vi "UHR-Fleezers Control (host) - 11.9.vi"() -> ()   [LabVIEW 2014] (continued)
            n1964 = Reshape Array(w2812, 3 ("dimension size")) -> (w2810:dbl[])
            n1965 = Array To Cluster(array=w2810) -> (cluster=w2809:cluster{"[0]":dbl, "[1]":dbl, "[2]":dbl})
            n1966 = call "Set Stage Position.vi"("Position"=w2809, "error in"=w2804, "VISA resource name in"=w2805) -> ("error out"=w2808:errorcluster)  [unwired: 2 out]
            n1967 = local write "Stage Moving"(TRUE ("Stage Moving")) -> ()
            n1968 = local write "Stage Control Serial Error"(w2808) -> ()
          }
          frame #1 {
            n1969 = local write "Stage Moving"(FALSE ("Stage Moving")) -> ()
            n1970 = call <vilib>:"Beep.vi"() -> ()  [unwired: 3 in, 9 out]
          }
        }
      }
      event "Set Current\nPos to 0,0,0": Value Change {
        # "DH is \"Define Home\""
        n1971 = event-data() -> ()  [unwired: 1 in, 6 out]
        n1972 = local write "Set Current\nPos to 0,0,0"(FALSE ("Set Current\nPos to 0,0,0")) -> ()
        n1973 = Concatenate Strings("1DH" ("string"), ";" ("string"), "2DH" ("string"), ";" ("string"), "3DH" ("string"), "\r") -> (w2823:string)
        n1974 = call-poly "VISA Configure Serial Port"("VISA resource name"=w2828, "baud rate (9600)"=u32 19200, "error in (no error)"=w2827) -> ("VISA resource name out"=w2825:refnum<visa-resource-name>, "error out"=w2824:errorcluster)  [unwired: 11 in]
        n1975 = VISA Write(VISA resource name=w2825, write buffer=w2823, error in (no error)=w2824) -> (error out=w2818:errorcluster)  [unwired: 2 out]
        n1976 = local write "Stage Control Serial Error"(w2818) -> ()
      }
      event "Got ADig bead": Value Change {
        n1977 = event-data() -> ()  [unwired: 1 in, 5 out]
        n1978 = flat-sequence {
          frame #0 {
            n1979 = local read "Cap 1 Samp Flow ON"() -> (w2833:bool)
            n1980 = case shown="True" w2833 {
              frame False {
              }
              frame True {
                n1981 = property on="Sample Channel\nFlow" class="Bool (strict)"("Val(Sgnl)"=TRUE ("Value (Signaling)")) -> ()  [unwired: 2 in, 2 out]
              }
            }
          }
          frame #1 {
            n1982 = property on="Inject Pump 3" class="Bool (strict)"("Val(Sgnl)"=FALSE ("Value (Signaling)")) -> ()  [unwired: 2 in, 2 out]
            n1983 = local write "Target"(FALSE ("Target")) -> ()
          }
          frame #2 {
            n1984 = property on="Move Cap. 1 (DNA Bottom)" class="Bool (strict)"("Val(Sgnl)"=TRUE ("Value (Signaling)")) -> ()  [unwired: 2 in, 2 out]
          }
        }
      }
      event "Force FB Script": Value Change {
        n1985 = event-data() -> ()  [unwired: 1 in, 5 out]
        n1986 = local write "Force FB Script"(FALSE ("Force FB Data\nScript")) -> ()
        n1987 = flat-sequence {
          tunnel: w2844 -> [w2848]
          tunnel: w2845 -> [w2849]
          tunnel: [w2849] -> w2840
          tunnel: [w2848] -> w2839
          tunnel: w2840 -> [w2852]
          tunnel: w2839 -> [w2851]
          tunnel: ["Trap Trig Fl."] -> w2841
          tunnel: [w2894] -> w2842
          tunnel: w2841 -> [w2894]
          tunnel: [w2898] -> w2843
          tunnel: w2842 -> [w2898]
          tunnel: w2843 -> [w2900]
          frame #0 {
            n1988 = property on="Trap D (MHz)" class="DigNum (strict)"("Val(Sgnl)"="Trap D Before Moving") -> ()  [unwired: 2 in, 2 out]
          }
          frame #1 {
            n1989 = local read "Saved Stage Positions"() -> (w2854:dbl[][])
            n1990 = local write "FB Trap Pos Offset"(0.0 ("FB Trap Pos Offset")) -> ()
            n1991 = property on="Trap Pos. FB Offset Factor" class="DigNum (strict)"("Val(Sgnl)"=i64 0 ("Value (Signaling)")) -> ()  [unwired: 2 in, 2 out]
            n1992 = local write "Stage Moving"(TRUE ("Stage Moving")) -> ()
            n1993 = call "move to saved stage position.vi"("error in"=w2851, "Stage VISA resource name in"=w2852, "Position"="Stage Position To Establish FB", "Saved Stage Positions"=w2854) -> ("error out"=w2850:errorcluster)  [unwired: 1 out]
            n1994 = local write "Stage Control Serial Error"(w2850) -> ()
          }
          frame #2 {
            n1995 = call <vilib>:"Beep.vi"("duration (msec)"=u32 100, "frequency (Hz)"=u32 20) -> ()  [unwired: 1 in, 9 out]
            n1996 = local write "Stage Moving"(FALSE ("Stage Moving")) -> ()
            n1997 = property on="Tab Control 2" class="TabCtl (strict)"("Val(Sgnl)"=T6."Feedback on Trap Position" ("Value (Signaling)")) -> ()  [unwired: 2 in, 2 out]
            n1998 = stacked-sequence {
              frame #0 {
                n1999 = Multiply(x="Wait (s)", y=u32 1000 ("milliseconds to wait")) -> (x*y=w2863:u32)
                n2000 = property on="Trap D (MHz)" class="DigNum (strict)"("Val(Sgnl)"="Starting Trap D (MHz)") -> ()  [unwired: 2 in, 2 out]
                n2001 = Wait (ms)(milliseconds to wait=w2863) -> ()  [unwired: 1 out]
              }
              frame #1 {
                n2002 = property on="Set Reading to\nSetpoint" class="Bool (strict)"("Val(Sgnl)"=TRUE ("Value (Signaling)")) -> ()  [unwired: 2 in, 2 out]
              }
            }
            n2003 = property on="Tab Control" class="TabCtl (strict)"("Val(Sgnl)"=T4."Trap Control (RF)" ("Value (Signaling)")) -> ()  [unwired: 2 in, 2 out]
          }
          frame #3 {
            n2004 = Wait (ms)(milliseconds to wait=u32 500) -> ()  [unwired: 1 out]
          }
          frame #4 {
            n2005 = property on="Trap Pos. FB ON" class="Bool (strict)"("Val(Sgnl)"=TRUE ("Value (Signaling)")) -> ()  [unwired: 2 in, 2 out]
            n2006 = Wait (ms)(milliseconds to wait=u32 250) -> ()  [unwired: 1 out]
          }
          frame #5 {
            n2007 = case shown="\"1\"" "Remove Action Offset Dropdown" {
              tunnel: TRUE ("Value (Signaling)") -> [w2875 w2883 w2891]
              frame "1" {
                n2008 = flat-sequence {
                  tunnel: w2875 -> [w2882]
                  frame #0 {
                    n2009 = local read "factor"() -> (w2877:dbl)
                    n2010 = Greater Than 0?(x=w2877) -> (x > 0?=w2881:bool)
                    n2011 = Select(t=1.0, s=w2881, f=-1.0) -> (s? t:f=w2878:dbl)
                    n2012 = Multiply(x=w2878, y=w2877) -> (x*y=w2876:dbl)
                    n2013 = local write "factor"(w2876) -> ()
                  }
                  frame #1 {
                    n2014 = property on="Remove Offset to factor" class="Bool (strict)"("Val(Sgnl)"=w2882) -> ()  [unwired: 2 in, 2 out]
                  }
                }
              }
              frame "2" {
                n2015 = flat-sequence {
                  tunnel: w2883 -> [w2890]
                  frame #0 {
                    n2016 = local read "factor"() -> (w2884:dbl)
                    n2017 = Greater Than 0?(x=w2884) -> (x > 0?=w2889:bool)
                    n2018 = Select(t=-1.0, s=w2889, f=1.0) -> (s? t:f=w2887:dbl)
                    n2019 = Multiply(x=w2884, y=w2887) -> (x*y=w2886:dbl)
                    n2020 = local write "factor"(w2886) -> ()
                  }
                  frame #1 {
                    n2021 = property on="Remove Offset to factor" class="Bool (strict)"("Val(Sgnl)"=w2890) -> ()  [unwired: 2 in, 2 out]
                  }
                }
              }
              frame "0", Default {
                n2022 = property on="Remove Action Offset" class="Bool (strict)"("Val(Sgnl)"=w2891) -> ()  [unwired: 2 in, 2 out]
              }
            }
            n2023 = case shown="False" "Trap Trig Fl." {
              frame False {
                n2024 = case shown="True" "Green ON after FB ON?" {
                  selector: "Green ON after FB ON?" -> [_ w2893]
                  frame False {
                  }
                  frame True {
                    n2025 = property on="Green ON/Interlacing" class="Bool (strict)"("Val(Sgnl)"=w2893) -> ()  [unwired: 2 in, 2 out]
                  }
                }
              }
              frame True {
              }
            }
            n2026 = Wait (ms)(milliseconds to wait=u32 250) -> ()  [unwired: 1 out]
          }
          frame #6 {
            n2027 = property on="Start Saving" class="Bool (strict)"("Val(Sgnl)"=TRUE ("Value (Signaling)")) -> ()  [unwired: 2 in, 2 out]
            n2028 = Wait (ms)(milliseconds to wait=u32 5000) -> ()  [unwired: 1 out]
          }
          frame #7 {
            w2897 = TRUE ("Value (Signaling)")
            n2029 = property on="Rem fb disp offset" class="Bool (strict)"("Val(Sgnl)"=w2897) -> ()  [unwired: 2 in, 2 out]
            n2030 = property on="Remove Offset" class="Bool (strict)"("Val(Sgnl)"=w2897) -> ()  [unwired: 2 in, 2 out]
            n2031 = Wait (ms)(milliseconds to wait=u32 100) -> ()  [unwired: 1 out]
          }
          frame #8 {
            n2032 = case shown="True" w2900 {
              frame False {
              }
              frame True {
                n2033 = local write "Trap Trig. Fl."(TRUE ("Value (Signaling)")) -> ()
              }
            }
          }
          frame #9 {
            n2034 = local read "Tether"() -> (w2903:bool)
            n2035 = And(x="Start dipping after?", y=w2903) -> (x .and. y?=w2902:bool)
            n2036 = case shown="True" w2902 {
              frame False {
              }
              frame True {
                n2037 = flat-sequence {
                  frame #0 {
                    n2038 = Multiply(x="Delay before dipping (s)", y=1000.0) -> (x*y=w2906:dbl)
                    n2039 = Wait (ms)(milliseconds to wait=w2906) -> ()  [unwired: 1 out]
                  }
                  frame #1 {
                    n2040 = property on="Dip for Protein" class="Bool (strict)"("Val(Sgnl)"=TRUE ("Value (Signaling)")) -> ()  [unwired: 2 in, 2 out]
                    n2041 = local write "Scripts"(T29."Dipping") -> ()
                  }
                }
              }
            }
          }
        }
      }
      event "Rupture Script": Value Change {
        n2042 = event-data() -> ()  [unwired: 1 in, 5 out]
        n2043 = local write "Rupture Script"(FALSE ("Rupture Script")) -> ()
        n2044 = flat-sequence {
          frame #0 {
            w2912 = TRUE
            w2917 = FALSE
            # "Number 6 for now is the\nrupture-experiment\nparameters."
            n2045 = local read "Starting Trap D (MHz)"() -> (w2918:dbl)
            n2046 = local write "Restart DMA? (AOD)"(w2917) -> ()
            n2047 = Replace Array Subset(array=u32[] [0] ("Index Values"), new element=6, index=0) -> (w2913:u32[])
            n2048 = local write "Save scans"(w2917) -> ()
            n2049 = property on="Trap D (MHz)" class="DigNum (strict)"("Val(Sgnl)"=w2918) -> ()  [unwired: 2 in, 2 out]
            n2050 = property on="Saved AOD Raster Scan Parameter Sets" class="Arr (strict)"("Index Values"=w2913) -> ()  [unwired: 2 in, 2 out]
            n2051 = property on="Start Saving" class="Bool (strict)"("Val(Sgnl)"=w2912) -> ()  [unwired: 2 in, 2 out]
            n2052 = property on="Green ON/Interlacing" class="Bool (strict)"("Val(Sgnl)"=w2912) -> ()  [unwired: 2 in, 2 out]
          }
          frame #1 {
            n2053 = property on="Load parameters" class="Bool (strict)"("Val(Sgnl)"=TRUE ("Value (Signaling)")) -> ()  [unwired: 2 in, 2 out]
          }
        }
      }
      event "Fixed Traps Script": Value Change {
        n2054 = event-data() -> ()  [unwired: 1 in, 5 out]
        n2055 = local write "Fixed Traps Script"(FALSE ("Fixed Traps Data\nScript")) -> ()
        n2056 = flat-sequence {
          frame #0 {
            n2057 = case shown="True" "Green ON" {
              frame False {
              }
              frame True {
                n2058 = property on="Green ON/Interlacing" class="Bool (strict)"("Val(Sgnl)"=TRUE) -> ()  [unwired: 2 in, 2 out]
              }
            }
            n2059 = local write "Offset (nm)"(0.0 ("Offset (nm)")) -> ()
            n2060 = property on="Sample Channel\nFlow" class="Bool (strict)"("Val(Sgnl)"=FALSE ("Value (Signaling)")) -> ()  [unwired: 2 in, 2 out]
            n2061 = property on="Trap D (MHz)" class="DigNum (strict)"("Val(Sgnl)"="Fixed Traps Trap Delta (MHz)") -> ()  [unwired: 2 in, 2 out]
          }
          frame #1 {
            n2062 = Wait (ms)(milliseconds to wait=u32 1000) -> ()  [unwired: 1 out]
          }
          frame #2 {
            n2063 = local write "Start Saving"(TRUE ("Start Saving")) -> ()
          }
          frame #3 {
            n2064 = local read "Bead Sep. Int. Time (s)"() -> (w2928:dbl)
            n2065 = Multiply(x=w2928, y=1000.0) -> (x*y=w2930:dbl)
            n2066 = Wait (ms)(milliseconds to wait=w2930) -> ()  [unwired: 1 out]
          }
          frame #4 {
            n2067 = property on="Remove Offset" class="Bool (strict)"("Val(Sgnl)"=TRUE ("Value (Signaling)")) -> ()  [unwired: 2 in, 2 out]
          }
          frame #5 {
            n2068 = property on="Dip for Protein" class="Bool (strict)"("Val(Sgnl)"="Start dipping after?") -> ()  [unwired: 2 in, 2 out]
          }
        }
      }
      event "Got DNA bead": Value Change {
        n2069 = event-data() -> ()  [unwired: 1 in, 5 out]
        n2070 = flat-sequence {
          frame #0 {
            n2071 = local read "Daq spot flow on"() -> (w2935:bool)
            n2072 = case shown="True" w2935 {
              frame False {
              }
              frame True {
                n2073 = property on="Sample Channel\nFlow" class="Bool (strict)"("Val(Sgnl)"=TRUE ("Value (Signaling)")) -> ()  [unwired: 2 in, 2 out]
              }
            }
            n2074 = property on="Got DNA bead" class="Bool"("Key Focus"=FALSE) -> ()  [unwired: 2 in, 2 out]
          }
          frame #1 {
            n2075 = property on="Inject Pump 1" class="Bool (strict)"("Val(Sgnl)"=FALSE ("Value (Signaling)")) -> ()  [unwired: 2 in, 2 out]
          }
          frame #2 {
            n2076 = property on="Cal/Data Acq. Spot" class="Bool (strict)"("Val(Sgnl)"=TRUE ("Value (Signaling)")) -> ()  [unwired: 2 in, 2 out]
          }
        }
      }
      event "Take Stepping Data": Value Change {
        n2077 = event-data() -> ()  [unwired: 1 in, 5 out]
        n2078 = local read "Save ave N"() -> (w2947:dbl)
        n2079 = flat-sequence {
          tunnel: w2947 -> [w2949]
          tunnel: [w2949] -> w2942
          tunnel: [w2951] -> w2943
          tunnel: w2942 -> [w2951]
          tunnel: [w2953] -> w2944
          tunnel: w2943 -> [w2953]
          tunnel: [w2956] -> w2945
          tunnel: w2944 -> [w2956]
          tunnel: [w2958] -> w2946
          tunnel: w2945 -> [w2958]
          tunnel: [w2960] -> w2940
          tunnel: w2946 -> [w2960]
          tunnel: w2940 -> [w2963]
          tunnel: [w2963] -> w2939
          tunnel: w2939 -> [w2964]
          tunnel: [w2964] -> w2941
          tunnel: w2941 -> [w2970]
          frame #0 {
            n2080 = property on="Save ave N" class="DigNum (strict)"("Val(Sgnl)"="Save ave factor") -> ()  [unwired: 2 in, 2 out]
          }
          frame #1 {
            n2081 = Wait (ms)(milliseconds to wait=u32 100) -> ()  [unwired: 1 out]
          }
          frame #2 {
            n2082 = local read "Offset 2 Start (MHz)"() -> (w2955:dbl)
            n2083 = property on="Saved AOD Raster Scan Parameter Sets" class="Arr (strict)"("Index Values"=u32[] [2]) -> ()  [unwired: 2 in, 2 out]
            n2084 = property on="Trap D (MHz)" class="DigNum (strict)"("Val(Sgnl)"=w2955) -> ()  [unwired: 2 in, 2 out]
          }
          frame #3 {
            n2085 = property on="Load parameters" class="Bool (strict)"("Val(Sgnl)"=TRUE ("Value (Signaling)")) -> ()  [unwired: 2 in, 2 out]
          }
          frame #4 {
            n2086 = Wait (ms)(milliseconds to wait=u32 100) -> ()  [unwired: 1 out]
          }
          frame #5 {
            n2087 = property on="Trap Raster Scan" class="Bool (strict)"("Val(Sgnl)"=TRUE ("Value (Signaling)")) -> ()  [unwired: 2 in, 2 out]
          }
          frame #6 {
            n2088 = Wait (ms)(milliseconds to wait=u32 1000) -> ()  [unwired: 1 out]
          }
          frame #7 {
            n2089 = while {
              stop <- w2967 stop-if-true
              n2090 = local read "Raster Scanning..."() -> (w2969:bool)
              n2091 = local read "Saving..."() -> (w2968:bool)
              n2092 = Not(x=w2968) -> (.not. x?=w2965:bool)
              n2093 = Not(x=w2969) -> (.not. x?=w2966:bool)
              n2094 = And(x=w2966, y=w2965) -> (x .and. y?=w2967:bool)
            }
          }
          frame #8 {
            n2095 = property on="Save ave N" class="DigNum (strict)"("Val(Sgnl)"=w2970) -> ()  [unwired: 2 in, 2 out]
          }
        }
      }
      event "Step Size (nm)": Value Change {
        n2096 = event-data() -> ()  [unwired: 1 in, 5 out]
        n2097 = flat-sequence {
          frame #0 {
            n2098 = property on="Saved AOD Raster Scan Parameter Sets" class="Arr (strict)"("Index Values"=u32[] [1]) -> ()  [unwired: 2 in, 2 out]
          }
          frame #1 {
            n2099 = Multiply(x="N Steps", y="Step Size (nm)") -> (x*y=w2972:dbl)
            n2100 = property on="Scan Speed AOD (nm/s) 2" class="DigNum (strict)"("Value"="Step Size (nm)") -> ()  [unwired: 2 in, 2 out]
            n2101 = property on="Step Size AOD (nm) 2" class="DigNum (strict)"("Value"="Step Size (nm)") -> ()  [unwired: 2 in, 2 out]
            n2102 = property on="Scan Range AOD (nm) 2" class="DigNum (strict)"("Value"=w2972) -> ()  [unwired: 2 in, 2 out]
          }
        }
      }
      event "Take Detection Laser\nImage": Value Change {
        n2103 = event-data() -> ()  [unwired: 1 in, 5 out]
        n2104 = flat-sequence {
          tunnel: [w3000] -> w2990
          tunnel: [w2999] -> w2983
          tunnel: [w2998] -> w2975
          tunnel: [w3003] -> w2991
          tunnel: w2990 -> [w3003]
          tunnel: [w3002] -> w2984
          tunnel: w2983 -> [w3002]
          tunnel: [w3001] -> w2976
          tunnel: w2975 -> [w3001]
          tunnel: [w3007] -> w2992
          tunnel: w2991 -> [w3007]
          tunnel: [w3006] -> w2985
          tunnel: w2984 -> [w3006]
          tunnel: [w3005] -> w2977
          tunnel: w2976 -> [w3005]
          tunnel: [w3013] -> w2993
          tunnel: w2992 -> [w3013]
          tunnel: [w3012] -> w2986
          tunnel: w2985 -> [w3012]
          tunnel: [w3011] -> w2978
          tunnel: w2977 -> [w3011]
          tunnel: [w3017] -> w2994
          tunnel: w2993 -> [w3017]
          tunnel: [w3016] -> w2987
          tunnel: w2986 -> [w3016]
          tunnel: [w3015] -> w2979
          tunnel: w2978 -> [w3015]
          tunnel: [w3021] -> w2995
          tunnel: w2994 -> [w3021]
          tunnel: [w3020] -> w2988
          tunnel: w2987 -> [w3020]
          tunnel: [w3019] -> w2980
          tunnel: w2979 -> [w3019]
          tunnel: [w3025] -> w2996
          tunnel: w2995 -> [w3025]
          tunnel: [w3024] -> w2989
          tunnel: w2988 -> [w3024]
          tunnel: [w3023] -> w2981
          tunnel: w2980 -> [w3023]
          tunnel: w2996 -> [w3031]
          tunnel: w2989 -> [w3030]
          tunnel: [w3028] -> w2982
          tunnel: w2981 -> [w3028]
          tunnel: w2982 -> [w3032]
          frame #0 {
            n2105 = local read "Green ON/Interlacing"() -> (w3000:bool)
            n2106 = local read "Green laser mode"() -> (w2999:enum32{"Laser ON", "Laser OFF", "Interlace"})
            n2107 = local read "Green FB On/Off"() -> (w2998:bool)
          }
          frame #1 {
            n2108 = property on="Green FB On/Off" class="Bool (strict)"("Val(Sgnl)"=FALSE ("Value (Signaling)")) -> ()  [unwired: 2 in, 2 out]
          }
          frame #2 {
            n2109 = property on="Green ON/Interlacing" class="Bool (strict)"("Val(Sgnl)"=TRUE ("Value (Signaling)")) -> ()  [unwired: 2 in, 2 out]
            n2110 = property on="Flip Green Filter" class="Bool (strict)"("Val(Sgnl)"=TRUE ("Value (Signaling)")) -> ()  [unwired: 2 in, 2 out]
            n2111 = property on="Green laser mode" class="RadioBtnsControl (strict)"("Val(Sgnl)"=enum32{"Laser ON", "Laser OFF", "Interlace"}."Laser ON" ("Value (Signaling)")) -> ()  [unwired: 2 in, 2 out]
          }
          frame #3 {
            n2112 = Wait (ms)(milliseconds to wait=u32 500) -> ()  [unwired: 1 out]
          }
          frame #4 {
            n2113 = property on="Confocal\nImage" class="Bool (strict)"("Val(Sgnl)"=TRUE ("Value (Signaling)")) -> ()  [unwired: 2 in, 2 out]
          }
          frame #5 {
            n2114 = Wait (ms)(milliseconds to wait=u32 2000) -> ()  [unwired: 1 out]
          }
          frame #6 {
            n2115 = while {
              stop <- w3026 stop-if-true
              n2116 = local read "Saving..."() -> (w3027:bool)
              n2117 = Not(x=w3027) -> (.not. x?=w3026:bool)
            }
          }
          frame #7 {
            n2118 = property on="Flip Green Filter" class="Bool (strict)"("Val(Sgnl)"=TRUE ("Value (Signaling)")) -> ()  [unwired: 2 in, 2 out]
            n2119 = property on="Green ON/Interlacing" class="Bool (strict)"("Val(Sgnl)"=w3031) -> ()  [unwired: 2 in, 2 out]
            n2120 = property on="Green laser mode" class="RadioBtnsControl (strict)"("Val(Sgnl)"=w3030) -> ()  [unwired: 2 in, 2 out]
          }
          frame #8 {
            n2121 = property on="Green FB On/Off" class="Bool (strict)"("Val(Sgnl)"=w3032) -> ()  [unwired: 2 in, 2 out]
          }
        }
      }
      event "Stop All": Value Change {
        n2122 = event-data() -> ()  [unwired: 1 in, 5 out]
        n2123 = local read "Stop All"() -> (w3033:bool)
      }
    }
    n2124 = node-c288() -> ()  [unwired: 1 in, 1 out]
  }
  n2125 = node-c288() -> (w112:T21)  [unwired: 4 out]
  n2126 = timed-loop "Mouse control: trap position (AOM deflection), set confocal spot from image" {
    tunnel: [w3035] -> w200
    tunnel: w20 -> [w3034]
    timing: w112 -> [_]
    timing-out: [_] -> w111
    stop <- w3035 stop-if-true
    n2127 = node-c288() -> ()  [unwired: 2 out]
    n2128 = event shown="[0] \"Pane\": Mouse Down" {
      selector: _ -> [_ _]
      dyn-events: _ -> [_ _]
      timeout: _ -> [_ _]
      tunnel: w3034 -> [w3038 _]
      event Mouse Down {
        n2129 = event-data() -> ("Time"=w3040:u32, "Coords"=w3039:T7, "Button"=w3041:u16)  [unwired: 6 out]
        n2130 = case shown="1" w3041 {
          tunnel: w3040 -> [_ _ w3180]
          tunnel: w3039 -> [_ w3046 w3178]
          tunnel: w3038 -> [_ _ w3176]
          frame 0, Default {
          }
          frame 1 {
            n2131 = property on="APD 2" class="ImageControl"() -> ("Displayed Image Position"=w3060:cluster{"Left":i32, "Top":i32})  [unwired: 2 in, 2 out]
            n2132 = control-ref of="Primary Video Display"() -> (w3053:refnum<vi>)
            n2133 = property on="APD 1" class="ImageControl"() -> ("Displayed Image Position"=w3089:cluster{"Left":i32, "Top":i32})  [unwired: 2 in, 2 out]
            n2134 = property on="Detection Laser X" class="ImageControl"() -> ("Displayed Image Position"=w3086:cluster{"Left":i32, "Top":i32})  [unwired: 2 in, 2 out]
            n2135 = property on="Detection Laser Y" class="ImageControl"() -> ("Displayed Image Position"=w3085:cluster{"Left":i32, "Top":i32})  [unwired: 2 in, 2 out]
            n2136 = property on="APD 2" class="ImageControl"() -> ("Displayed Image Size"=w3059:cluster{"Width":u32, "Height":u32})  [unwired: 2 in, 2 out]
            n2137 = property on="APD 1" class="ImageControl"() -> ("Displayed Image Size"=w3087:cluster{"Width":u32, "Height":u32})  [unwired: 2 in, 2 out]
            n2138 = property on="Detection Laser X" class="ImageControl"() -> ("Displayed Image Size"=w3088:cluster{"Width":u32, "Height":u32})  [unwired: 2 in, 2 out]
            n2139 = property on="Detection Laser Y" class="ImageControl"() -> ("Displayed Image Size"=w3084:cluster{"Width":u32, "Height":u32})  [unwired: 2 in, 2 out]
            n2140 = property class="ImageControl"(reference=w3053) -> ("Displayed Image Position"=w3051:cluster{"Left":i32, "Top":i32})  [unwired: 1 in, 2 out]
            n2141 = property class="ImageControl"(reference=w3053) -> ("Displayed Image Size"=w3052:cluster{"Width":u32, "Height":u32})  [unwired: 1 in, 2 out]
            n2142 = Unbundle By Name(w3059) -> ("Width"=w3056:u32, "Height"=w3055:u32)
            n2143 = Unbundle By Name(w3060) -> ("Left"=w3058:i32, "Top"=w3057:i32)
            n2144 = Unbundle By Name(w3087) -> ("Width"=w3081:u32, "Height"=w3080:u32)
            n2145 = Unbundle By Name(w3088) -> ("Width"=w3077:u32, "Height"=w3076:u32)
            n2146 = Unbundle By Name(w3084) -> ("Width"=w3073:u32, "Height"=w3072:u32)
            n2147 = Unbundle By Name(w3089) -> ("Left"=w3083:i32, "Top"=w3082:i32)
            n2148 = Unbundle By Name(w3086) -> ("Left"=w3079:i32, "Top"=w3078:i32)
            n2149 = Unbundle By Name(w3085) -> ("Left"=w3075:i32, "Top"=w3074:i32)
            n2150 = Bundle("Left"=w3058, "Top"=w3057, "Width"=w3056, "Height"=w3055) -> (w3054:T30)  [unwired: 1 in]
            n2151 = Bundle("Left"=w3083, "Top"=w3082, "Width"=w3081, "Height"=w3080) -> (w3071:T30)  [unwired: 1 in]
            n2152 = Bundle("Left"=w3079, "Top"=w3078, "Width"=w3077, "Height"=w3076) -> (w3070:T30)  [unwired: 1 in]
            n2153 = Bundle("Left"=w3075, "Top"=w3074, "Width"=w3073, "Height"=w3072) -> (w3069:T30)  [unwired: 1 in]
            n2154 = Unbundle By Name(w3052) -> ("Width"=w3048:u32, "Height"=w3047:u32)
            n2155 = Unbundle By Name(w3051) -> ("Left"=w3050:i32, "Top"=w3049:i32)
            n2156 = Build Cluster Array(w3054, w3071, w3070, w3069) -> (w3068:T31)
            n2157 = Bundle("Left"=w3050, "Top"=w3049, "Width"=w3048, "Height"=w3047) -> (w3043:T30)  [unwired: 1 in]
            n2158 = for {
              tunnel: w3046 -> [w3122]
              tunnel: w3068 -> [w3123] mode=indexing
              shift-right: [w3120] -> w3066
              shift-left: TRUE -> [w3121]
              shift-right: [w3119] -> w3064
              shift-left: _ -> [w3115]
              shift-right: [w3118] -> w3063
              shift-left: _ -> [w3114]
              shift-right: [w3117] -> w3062
              shift-left: _ -> [w3113]
              shift-right: [w3116] -> w3061
              shift-left: _ -> [w3112]
              n2159 = case shown="True" w3121 {
                selector: w3121 -> [w3128 _]
                tunnel: w3123 -> [_ w3137]
                tunnel: w3122 -> [_ w3135]
                tunnel: [w3128 w3133] -> w3120
                tunnel: [w3127 w3132] -> w3119
                tunnel: [w3126 w3131] -> w3118
                tunnel: [w3125 w3130] -> w3117
                tunnel: [w3124 w3129] -> w3116
                tunnel: w3115 -> [w3127 _]
                tunnel: w3114 -> [w3126 _]
                tunnel: w3113 -> [w3125 _]
                tunnel: w3112 -> [w3124 _]
                frame False {
                }
                frame True {
                  n2160 = Unbundle(w3137) -> (w3136:T30)
                  n2161 = call "isclickinwindow.vi"("Image Param"=w3136, "Point32"=w3135) -> ("4 Y"=w3129:i32, "3 Height"=w3130:i32, "2 X"=w3131:i32, "1 Width"=w3132:i32, "In image?"=w3134:bool)  [unwired: 1 in]
                  n2162 = Not(x=w3134) -> (.not. x?=w3133:bool)
                }
              }
            }
            n2163 = call "isclickinwindow.vi"("Image Param"=w3043, "Point32"=w3046) -> ("4 Y"=w3044:i32, "2 X"=w3045:i32, "In image?"=w3042:bool)  [unwired: 1 in, 2 out]
            n2164 = case shown="True" w3042 {
              tunnel: w3045 -> [_ w3093]
              tunnel: w3044 -> [_ w3096]
              frame False {
              }
              frame True {
                w3105 = 2
                n2165 = Subtract(x=480, y=w3096) -> (x-y=w3095:i32)
                n2166 = Unbundle("Target size") -> ("Width"=w3106:dbl, "Height"=w3104:dbl)
                n2167 = Subtract(x=w3093, y=2) -> (x-y=w3092:i32)
                n2168 = Divide(x=w3104, y=w3105) -> (x/y=w3102:dbl)
                n2169 = Divide(x=w3106, y=w3105) -> (x/y=w3103:dbl)
                n2170 = Subtract(x=w3092, y=w3103) -> (x-y=w3101:dbl)
                n2171 = Add(x=w3092, y=w3103) -> (x+y=w3099:dbl)
                n2172 = Subtract(x=w3095, y=w3102) -> (x-y=w3100:dbl)
                n2173 = Add(x=w3095, y=w3102) -> (x+y=w3098:dbl)
                n2174 = Bundle(w3092, w3095) -> (w3108:cluster{i32, i32})  [unwired: 1 in]
                n2175 = Bundle(w3101, w3100, w3099, w3098) -> (w3090:cluster{dbl, dbl, dbl, dbl})  [unwired: 1 in]
                n2176 = case shown="True" "Set target" {
                  tunnel: w3108 -> [_ w3111]
                  tunnel: w3090 -> [_ w3109]
                  frame False {
                  }
                  frame True {
                    n2177 = local write "Target coordinates"(w3109) -> ()
                    n2178 = local write "Set target"(FALSE ("Set target")) -> ()
                    "Video coordinates" <- w3111
                  }
                }
              }
            }
            n2179 = Not(x=w3066) -> (.not. x?=w3065:bool)
            n2180 = case shown="True" w3065 {
              tunnel: w3063 -> [_ w3151]
              tunnel: w3061 -> [_ w3150]
              tunnel: w3064 -> [_ w3149]
              tunnel: w3062 -> [_ w3148]
              frame False {
              }
              frame True {
                w3138 = FALSE ("Get Point")
                n2181 = local read "Scan lines (y)"() -> (w3153:u64)
                n2182 = disable-structure shown="Disabled" {
                  frame Disabled {
                  }
                  frame Enabled {
                  }
                }
                n2183 = local read "Actual MCL Inc (V)"() -> (w3147:dbl)
                n2184 = local read "Scan steps (MCL)"() -> (w3152:u64)
                n2185 = Divide "Y Pix/step"(x=w3148, y=w3153) -> (x/y=w3160:dbl)
                n2186 = Divide "Y V/pix"(x=w3147, y=w3160) -> (x/y=w3159:dbl)
                n2187 = Divide "Y half step offset"(x=w3147, y=2.0) -> (x/y=w3161:dbl)
                n2188 = Divide "X pix/step"(x=w3149, y=w3152) -> (x/y=w3158:dbl)
                n2189 = Negate(x=w3161) -> (-x=w3162:dbl)
                n2190 = local read "Initial Y"() -> (w3168:dbl)
                n2191 = Multiply(x=w3150, y=w3159) -> (x*y=w3169:dbl)
                n2192 = Divide "X half step offset"(x=w3147, y=2.0) -> (x/y=w3155:dbl)
                n2193 = Divide "X V/pix"(x=w3147, y=w3158) -> (x/y=w3157:dbl)
                n2194 = Multiply(x=w3147, y=w3152) -> (x*y=w3164:dbl)
                n2195 = Compound Arithmetic op=ADD(w3162, w3169, w3168) -> (w3139:dbl)
                "Pointer Y (V)" <- w3139
                n2196 = Multiply(x=w3157, y=w3151) -> (x*y=w3166:dbl)
                n2197 = Negate(x=w3155) -> (-x=w3154:dbl)
                n2198 = local read "Initial X"() -> (w3167:dbl)
                n2199 = Negate(x=w3166) -> (-x=w3165:dbl)
                n2200 = Compound Arithmetic op=ADD(w3154, w3164, w3167, w3165) -> (w3140:dbl)
                "Pointer X (V)" <- w3140
                n2201 = case shown="True" "Set High F Confocal Spot (X-Y)" {
                  tunnel: w3140 -> [_ w3170]
                  tunnel: w3139 -> [_ w3171]
                  frame False {
                  }
                  frame True {
                    "Confocal Y 2 (V)" <- w3171
                    "Confocal X 2 (V)" <- w3170
                  }
                }
                n2202 = Or(x="Set X Only", y="Set Confocal Spot (X-Y)") -> (x .or. y?=w3143:bool)
                n2203 = Or(x="Set Confocal Spot (X-Y)", y="Set Y Only") -> (x .or. y?=w3142:bool)
                n2204 = case shown="True" w3143 {
                  tunnel: w3140 -> [_ w3172]
                  frame False {
                  }
                  frame True {
                    n2205 = property on="AO2" class="Slide (strict)"("Val(Sgnl)"=w3172) -> ()  [unwired: 2 in, 2 out]
                    "Confocal X 1 (V)" <- w3172
                  }
                }
                n2206 = case shown="True" w3142 {
                  tunnel: w3139 -> [_ w3173]
                  frame False {
                  }
                  frame True {
                    n2207 = property on="AO1" class="Slide (strict)"("Val(Sgnl)"=w3173) -> ()  [unwired: 2 in, 2 out]
                    "Confocal Y 1 (V)" <- w3173
                  }
                }
                n2208 = local write "Set High F Confocal Spot (X-Y)"(w3138) -> ()
                n2209 = local write "Set Confocal Spot (X-Y)"(w3138) -> ()
                n2210 = local write "Set X Only"(w3138) -> ()
                n2211 = local write "Set Y Only"(w3138) -> ()
              }
            }
          }
          frame 3 {
            n2212 = local read "BD 2 Frequency 1 (MHz)"() -> (w3174:dbl)
            n2213 = local read "BD 1 Frequency 1 (MHz)"() -> (w3175:dbl)
            n2214 = local write "Manipulating Trap"(TRUE ("Manipulating Trap")) -> ()
            n2215 = local write "Coords"(T7 {"Horizontal"=0, "Vertical"=0} ("Coords")) -> ()
            n2216 = while {
              tunnel: w3180 -> [w3185]
              tunnel: w3178 -> [w3184]
              tunnel: w3176 -> [w3183]
              tunnel: w3175 -> [w3182]
              tunnel: w3174 -> [w3181]
              stop <- w3186 stop-if-true
              n2217 = event shown="[0] \"Pane\": Mouse Move" {
                selector: _ -> [_ _]
                dyn-events: _ -> [_ _]
                timeout: _ -> [_ _]
                tunnel: ["Force Manip Abort" w3250] -> w3186
                tunnel: w3185 -> [w3193 _]
                tunnel: w3184 -> [w3191 _]
                tunnel: w3183 -> [w3190 _]
                tunnel: w3182 -> [w3189 _]
                tunnel: w3181 -> [w3188 _]
                event Mouse Move {
                  n2218 = event-data() -> ("Time"=w3194:u32, "Coords"=w3195:T7)  [unwired: 3 out]
                  n2219 = Less?(x=w3194, y=w3193) -> (x < y?=w3192:bool)
                  n2220 = case "Makes sure old motion events prior to mouse click aren't used" shown="False" w3192 {
                    tunnel: w3195 -> [w3237 _]
                    tunnel: w3191 -> [w3238 _]
                    tunnel: w3190 -> [w3215 _]
                    tunnel: w3189 -> [w3211 _]
                    tunnel: w3188 -> [w3210 _]
                    frame False {
                      n2221 = Subtract(x=w3237, y=w3238) -> (x-y=w3236:T7)
                      "Coords" <- w3236
                      n2222 = local read "Y RF Frequency Limits (MHz)"() -> (w3196:T16)
                      n2223 = To Double Precision Float(number=w3236) -> (double precision float=w3235:cluster{"Horizontal":dbl, "Vertical":dbl})
                      n2224 = Multiply(x=cluster{"Horizontal":dbl, "Vertical":dbl} {"Horizontal"=-1.0, "Vertical"=1.0}, y="Manipulation Scaling") -> (x*y=w3231:cluster{"Horizontal":dbl, "Vertical":dbl})
                      n2225 = local read "X RF Frequency Limits (MHz)"() -> (w3197:T16)
                      n2226 = Multiply(x=w3235, y=w3231) -> (x*y=w3233:cluster{"Horizontal":dbl, "Vertical":dbl})
                      n2227 = Unbundle By Name(w3233) -> ("Horizontal"=w3228:dbl, "Vertical"=w3232:dbl)
                      n2228 = Unbundle By Name(w3196) -> ("Maximum"=w3199:dbl, "Minimum"=w3198:dbl)
                      n2229 = Boolean To (0,1)(Boolean="Manip. X?") -> (0, 1=w3226:i16)
                      n2230 = Boolean To (0,1)(Boolean="Manip. Y?") -> (0, 1=w3223:i16)
                      n2231 = local read "BD 1 Frequency 2 (MHz)"() -> (w3213:dbl)
                      n2232 = Multiply(x=w3232, y=w3223) -> (x*y=w3225:dbl)
                      n2233 = Multiply(x=w3226, y=w3228) -> (x*y=w3229:dbl)
                      n2234 = local read "BD 2 Frequency 2 (MHz)"() -> (w3212:dbl)
                      n2235 = Unbundle By Name(w3197) -> ("Maximum"=w3201:dbl, "Minimum"=w3200:dbl)
                      n2236 = Add(x=w3210, y=w3225) -> (x+y=w3203:dbl)
                      n2237 = Add(x=w3211, y=w3229) -> (x+y=w3205:dbl)
                      n2238 = In Range and Coerce(upper limit=w3201, x=w3205, lower limit=w3200) -> (coerced(x)=w3204:dbl)  [unwired: 1 out]
                      n2239 = In Range and Coerce(upper limit=w3199, x=w3203, lower limit=w3198) -> (coerced(x)=w3202:dbl)  [unwired: 1 out]
                      n2240 = Subtract(x=w3204, y=w3213) -> (x-y=w3222:dbl)
                      n2241 = Subtract(x=w3202, y=w3212) -> (x-y=w3221:dbl)
                      n2242 = Square(x=w3222) -> (x^2=w3220:dbl)
                      n2243 = Square(x=w3221) -> (x^2=w3219:dbl)
                      n2244 = Add(x=w3220, y=w3219) -> (x+y=w3218:dbl)
                      n2245 = Square Root(x=w3218) -> (sqrt(x)=w3214:dbl)
                      n2246 = In Range and Coerce(upper limit="Limit Max (MHz)", x=w3214, lower limit="Limit Min (MHz)") -> (In Range?=w3207:bool)  [unwired: 1 out]
                      n2247 = Not(x="Limits Enable") -> (.not. x?=w3206:bool)
                      n2248 = Or(x=w3207, y=w3206) -> (x .or. y?=w3208:bool)
                      n2249 = case shown="True" w3208 {
                        tunnel: w3215 -> [_ w3248]
                        tunnel: w3214 -> [_ w3239]
                        tunnel: w3204 -> [_ w3246]
                        tunnel: w3213 -> [_ w3245]
                        tunnel: w3202 -> [_ w3244]
                        tunnel: w3212 -> [_ w3243]
                        tunnel: w3197 -> [_ w3241]
                        tunnel: w3196 -> [_ w3240]
                        frame False {
                        }
                        frame True {
                          n2250 = local read "BD 1 Frequency 3 (MHz)"() -> (w3247:dbl)
                          n2251 = local read "BD 2 Frequency 3 (MHz)"() -> (w3242:dbl)
                          n2252 = local write "Trap D (MHz)"(w3239) -> ()
                          n2253 = call "set RF board frequency - interlace.vi"("Board 2 Frequency Limits"=w3240, "Board 1 Frequency Limits"=w3241, "FPGA VI Reference In"=w3248, "Board 2 Frequency 3 (MHz)"=w3242, "Board 1 Frequency 3 (MHz)"=w3247, "Board 2 Frequency 2 (MHz)"=w3243, "Board 2 Frequency 1 (MHz)"=w3244, "Board 1 Frequency 2 (MHz)"=w3245, "Board 1 Frequency 1  (MHz)"=w3246) -> ()  [unwired: 1 in, 2 out]
                          n2254 = local write "BD 2 Frequency 1 (MHz)"(w3244) -> ()
                          n2255 = local write "BD 1 Frequency 1 (MHz)"(w3246) -> ()
                        }
                      }
                    }
                    frame True {
                    }
                  }
                }
                event Mouse Up {
                  n2256 = event-data() -> ("Button"=w3249:u16)  [unwired: 8 out]
                  n2257 = case shown="3" w3249 {
                    tunnel: [FALSE TRUE] -> w3250
                    frame 0, Default {
                    }
                    frame 3 {
                      n2258 = local read "Trap D (MHz)"() -> (w3252:dbl)
                      n2259 = property on="Initial D (MHz)" class="DigNum (strict)"("Val(Sgnl)"=w3252) -> ()  [unwired: 2 in, 2 out]
                      n2260 = local write "Manipulating Trap"(FALSE ("Manipulating Trap")) -> ()
                    }
                  }
                }
              }
            }
          }
        }
      }
      event Mouse Move {
        n2261 = event-data() -> ()  [unwired: 6 out]
      }
    }
    n2262 = local read "Stop All"() -> (w3035:bool)
    n2263 = node-c288() -> ()  [unwired: 2 out]
  }
  n2264 = node-c288(w109) -> ()  [unwired: 1 out]
  n2265 = node-c288(w111) -> ()  [unwired: 1 out]
  n2266 = node-c288(w97) -> ()  [unwired: 1 out]
  n2267 = flat-sequence "Video" {
    tunnel: [w3263] -> w99
    tunnel: w99 -> [w3304]
    frame #0 {
      n2268 = while {
        stop <- w3256 continue-if-true
        n2269 = call "Close Video Capture.vi"() -> ("error code OUT"=w3258:i32)
        n2270 = Equal?(x=w3258, y=0) -> (x = y?=w3256:bool)
      }
      n2271 = local write "Stop All"(FALSE ("Stop All")) -> ()
    }
    frame #1 {
      n2272 = call "DMR_Init.vi"() -> ()  [unwired: 3 out]
    }
    frame #2 {
      # "Setting the destination format to Mono8 makes sure that the image can be displayed in the intensity plot."
      n2273 = call "DMR_GetDevice.vi"("search string IN"="DE019116701") -> ("device handle OUT"=w3281:i32)  [unwired: 4 in, 2 out]
      n2274 = call "DMR_OpenDevice.vi"("device handle IN"=w3281) -> ("driver handle OUT"=w3264:i32)  [unwired: 4 out]
      n2275 = call "DMR_FindList.vi"("flags IN"=u32 0 ("flags"), "list name IN"="" ("String"), "list type IN"=T32."camera descriptions", "driver handle IN"=w3264) -> ("list handle OUT"=w3267:i32)  [unwired: 2 out]
      n2276 = call "DMR_FindList.vi"("flags IN"=u32 0 ("flags"), "list name IN"="Base", "list type IN"=T32."setting", "driver handle IN"=w3264) -> ("list handle OUT"=w3265:i32)  [unwired: 2 out]
      n2277 = call "OBJ_GetHandle.vi"("object name IN"="VideoStandard", "list handle IN"=w3267) -> ("object handle OUT"=w3261:i32)  [unwired: 3 out]
      n2278 = call "OBJ_GetHandle.vi"("object name IN"="PixelFormat", "list handle IN"=w3265) -> ("object handle OUT"=w3275:i32)  [unwired: 3 out]
      n2279 = call "OBJ_SetS.vi"("value index IN"=0, "value IN"="NTSC M", "object handle IN"=w3261) -> ()  [unwired: 2 out]
      n2280 = call "OBJ_SetS.vi"("value index IN"=0, "value IN"="Mono8" ("value"), "object handle IN"=w3275) -> ()  [unwired: 2 out]
      n2281 = call "OBJ_GetHandle.vi"("object name IN"="VideoChannel", "list handle IN"=w3265) -> ("object handle OUT"=w3271:i32)  [unwired: 3 out]
      n2282 = while {
        tunnel: [w3286] -> w3263
        tunnel: w3264 -> [w3283]
        stop <- w3284 continue-if-true
        n2283 = call "DMR_ImageRequestSingle.vi"("request control IN"=0, "driver handle IN"=w3283) -> ("error code OUT"=w3285:i32, "driver handle OUT"=w3286:i32)  [unwired: 2 out]
        n2284 = Equal To 0?(x=w3285) -> (x = 0?=w3284:bool)
      }
      n2285 = call "OBJ_SetI.vi"("value index IN"=0, "value IN"=3 ("Video channel"), "object handle IN"=w3271) -> ()  [unwired: 2 out]
    }
    frame #3 {
      w3292 = T17 0 items=["Grayscale (U8)", "Grayscale (I16)", "Grayscale (SGL)", "Complex (CSG)", "RGB (U32)", "HSL (U32)", "RGB (U64)"] ("Image Type")
      w3300 = T17 0 items=["Grayscale (U8)", "Grayscale (I16)", "Grayscale (SGL)", "Complex (CSG)", "RGB (U32)", "HSL (U32)", "RGB (U64)"] ("Image Type")
      n2286 = for "Create Greyscale map" {
        N: 256 -> [_]
        tunnel: [w3306] -> w3289 mode=indexing
        workers-P: _ -> [_]
        i -> [w3309]
        n2287 = To Unsigned Byte Integer(number=w3309) -> (unsigned 8bit integer=w3305:u8)
        n2288 = Join Numbers(hi=w3305, lo=w3305) -> ((hi.lo)=w3308:u16)
        n2289 = Join Numbers(hi=w3305, lo=w3305) -> ((hi.lo)=w3307:u16)
        n2290 = Join Numbers(hi=w3308, lo=w3307) -> ((hi.lo)=w3306:u32)
      }
      n2291 = call "IMAQ Create"("Image Name"="Scaled video", "Image Type"=w3292) -> ("New Image"=w3291:T2)  [unwired: 2 in, 2 out]
      n2292 = call "IMAQ Create"("Image Name"="Main video", "Image Type"=w3300) -> ("New Image"=w3301:T2)  [unwired: 2 in, 2 out]
      n2293 = node-c288(0 ("Processor")) -> (w3299:T21)  [unwired: 3 out]
      n2294 = Initialize Array(u32 0 ("Window Number (0...15)"), 480 ("dimension size"), 640 ("dimension size")) -> (w3294:u32[][])
      n2295 = timed-loop {
        tunnel: w3304 -> [w3326]
        tunnel: [w3325] -> w3303
        tunnel: w3301 -> [w3324]
        timing: w3299 -> [_]
        timing-out: [_] -> w3298
        tunnel: w3294 -> [w3313]
        tunnel: w3291 -> [w3311]
        tunnel: w3289 -> [w3310]
        stop <- w3312 stop-if-true
        # "This block performs the \nactual image capture."
        n2296 = node-c288() -> ()  [unwired: 2 out]
        n2297 = local read "Stop All"() -> (w3312:bool)
        n2298 = Reciprocal(x="Video Capture Rate (Hz)") -> (1/x=w3316:dbl)
        n2299 = Multiply(x=w3316, y=1000.0) -> (x*y=w3314:dbl)
        n2300 = call "DMR_ImageRequestWaitFor.vi"("queue number IN"=0, "timeout(ms) IN"=500, "driver handle IN"=w3326) -> ("error code OUT"=w3330:i32, "request number OUT"=w3327:i32, "driver handle OUT"=w3328:i32)
        n2301 = feedback #1(T33 refnum ("Avi Refnum")) -> (w3318:T33)
        n2302 = case shown="True" "New Video File" {
          tunnel: [T33 refnum ("Avi Refnum") w3347] -> w3320
          tunnel: [FALSE TRUE] -> w3321
          tunnel: w3318 -> [_ w3343]
          frame False {
          }
          frame True {
            n2303 = call "Create new save file.vi"("Ext"=".avi" ("string"), "Index In"="Video Index") -> ("Path Out"=w3339:path, "Index Out"=w3340:dbl)  [unwired: 1 in]
            "Path Out" <- w3339
            n2304 = Not Equal?(x=w3343, y=T33 refnum ("Avi Refnum")) -> (x != y?=w3344:bool)
            n2305 = Increment(x=w3340) -> (x+1=w3349:dbl)
            n2306 = case shown="True" w3344 {
              tunnel: w3343 -> [_ w3350]
              frame False {
              }
              frame True {
                n2307 = call "IMAQ AVI Close"("Avi Refnum"=w3350) -> ()  [unwired: 1 in, 10 out]
              }
            }
            n2308 = local write "Video Index"(w3349) -> ()
            n2309 = call "IMAQ AVI Create"("Frames Per Second"=u32 30, "AVI Path"=w3339) -> ("Avi Refnum"=w3347:T33)  [unwired: 5 in, 4 out]
          }
        }
        n2310 = Equal To 0?(x=w3330) -> (x = 0?=w3329:bool)
        n2311 = Select(t=w3320, s=w3321, f=w3318) -> (s? t:f=w3319:T33)
        n2312 = feedback-in #1(w3319) -> ()
        n2313 = case shown="True" w3329 {
          tunnel: w3328 -> [w3351 w3378]
          tunnel: w3327 -> [_ w3377]
          tunnel: [w3351 w3374] -> w3325
          tunnel: w3324 -> [_ w3355]
          tunnel: w3313 -> [_ w3362]
          tunnel: w3319 -> [_ w3360]
          tunnel: w3311 -> [_ w3356]
          tunnel: w3310 -> [_ w3357]
          frame False {
          }
          frame True {
            w3368 = u32 0 ("X-offset IN")
            n2314 = call "DMR_GetImageRequestBufferData.vi"("driver handle IN"=w3378, "request number IN"=w3377) -> ("width OUT"=w3367:i32, "height OUT"=w3366:i32, "driver handle OUT"=w3373:i32, "request number OUT"=w3372:i32, "bytes per pixel OUT"=w3369:i32)  [unwired: 13 out]
            n2315 = call "DMR_GetImageRequestBufferImageData.vi"("driver handle IN"=w3373, "request number IN"=w3372, "bytes per pixel IN"=w3369, "X-offset IN"=w3368, "Y-offset IN"=w3368, "height IN"=w3366, "width IN"=w3367) -> ("driver handle OUT"=w3371:u32, "request number OUT"=w3370:u32, "image OUT"=w3363:u32[][])  [unwired: 10 out]
            n2316 = call "DMR_ImageRequestUnlock.vi"("request number IN"=w3370, "driver handle IN"=w3371) -> ("driver handle OUT"=w3376:i32)  [unwired: 1 in, 2 out]
            n2317 = case shown="True" "Averaging" {
              tunnel: w3363 -> [w3419 w3424]
              tunnel: [w3419 w3423] -> w3359
              tunnel: w3362 -> [_ w3421]
              frame False {
              }
              frame True {
                (unwired) 1
                w3429 = 1
                n2318 = feedback #2(w3421) -> (w3420:u32[][])
                n2319 = Add(x=w3424, y=w3420) -> (x+y=w3425:u32[][])
                n2320 = Select(t=w3421, s="Reset Averaging", f=w3425) -> (s? t:f=w3427:u32[][])
                n2321 = feedback-in #2(w3427) -> ()
                n2322 = feedback #3(w3429) -> (w3422:i32)
                n2323 = Divide(x=w3425, y=w3422) -> (x/y=w3426:dbl[][])
                n2324 = Increment(x=w3422) -> (x+1=w3430:i32)
                n2325 = To Unsigned Long Integer(number=w3426) -> (unsigned 32bit integer=w3423:u32[][])
                n2326 = Select(t=w3429, s="Reset Averaging", f=w3430) -> (s? t:f=w3428:i32)
                n2327 = feedback-in #3(w3428) -> ()
              }
            }
            n2328 = call "DMR_ImageRequestSingle.vi"("request control IN"=0, "driver handle IN"=w3376) -> ("driver handle OUT"=w3374:i32)  [unwired: 3 out]
            n2329 = disable-structure shown="Disabled" {
              disable-tunnel: w3359 -> [w3396 _]
              disable-tunnel: w3356 -> [w3395 _]
              frame Disabled {
                n2330 = To Double Precision Float(number=w3396) -> (double precision float=w3394:dbl[][])
                n2331 = In Range and Coerce(upper limit="Intensity Upper", x=w3394, lower limit="Intensity Lower") -> (coerced(x)=w3393:dbl[][])  [unwired: 1 out]
                n2332 = Subtract(x="Intensity Upper", y="Intensity Lower") -> (x-y=w3390:dbl)
                n2333 = Subtract(x=w3393, y="Intensity Lower") -> (x-y=w3391:dbl[][])
                n2334 = Divide(x=w3391, y=w3390) -> (x/y=w3392:dbl[][])
                n2335 = Multiply(x=255.0, y=w3392) -> (x*y=w3388:dbl[][])
                n2336 = To Unsigned Byte Integer(number=w3388) -> (unsigned 8bit integer=w3397:u8[][])
                n2337 = call "IMAQ ArrayToImage"("Image Pixels (U8)"=w3397, "Image"=w3395) -> ("Image Out"=w3384:T2)  [unwired: 4 in, 5 out]
                n2338 = First Call?() -> (First Call?: T/F=w3385:bool)
                n2339 = case shown="True" w3385 {
                  tunnel: w3384 -> [w3398 w3409]
                  frame False {
                    n2340 = flat-sequence {
                      tunnel: w3398 -> [w3404]
                      frame #0 {
                        w3401 = FALSE ("Get/Set Status? (Set)")
                        w3400 = 0 ("Window Number (0...15)")
                        n2341 = call "IMAQ WindSize"("Get/Set Status? (Set)"=w3401, "Window Number"=w3400) -> ("Width & Height out"=→"Window Size":cluster{"Width":i32, "Height":i32})  [unwired: 4 in, 2 out]
                        n2342 = call "IMAQ WindMove"("Window Number (0...15)"=w3400, "Get/Set Status? (Set)"=w3401) -> ("Coordinates (screen)"=→"Window Position":cluster{"X Position":i32, "Y Position":i32})  [unwired: 3 in, 1 out]
                        n2343 = call "IMAQ WindDraw"("Resize to Image Size? (Y)"=FALSE, "Window Number (0...15)"=w3400, "Image"=w3404) -> ()  [unwired: 7 in, 2 out]
                      }
                      frame #1 {
                        n2344 = call "IMAQ WindZoom 2"("Center Point"="Center Point", "Zoom to Fit? (False)"=FALSE, "Zoom Factor"="Zoom Factor") -> ()  [unwired: 5 in, 4 out]
                      }
                    }
                  }
                  frame True {
                    n2345 = flat-sequence {
                      tunnel: w3409 -> [w3412]
                      tunnel: [w3410] -> w3408
                      tunnel: w3408 -> [w3414]
                      frame #0 {
                        w3411 = TRUE ("Resize to Image Size? (Y)")
                        w3410 = 0 ("Window Number (0...15)")
                        n2346 = call "IMAQ WindNonTearing"("Window Number"=w3410, "NonTearing? (True)"=w3411) -> ()  [unwired: 8 in, 2 out]
                        n2347 = call "IMAQ WindDraw"("Resize to Image Size? (Y)"=w3411, "Window Number (0...15)"=w3410, "Image"=w3412) -> ()  [unwired: 7 in, 2 out]
                      }
                      frame #1 {
                        n2348 = call "IMAQ WindSize"("Scrollbars? (N)"=FALSE, "Width & Height"="Initial Window Size", "Window Number"=w3414) -> ()  [unwired: 3 in, 3 out]
                        n2349 = call "IMAQ WindMove"("Window Number (0...15)"=w3414, "Coordinates (screen)"="Initial Window Position") -> ()  [unwired: 3 in, 2 out]
                      }
                    }
                  }
                }
              }
              frame Enabled {
              }
            }
            n2350 = To Unsigned Byte Integer(number=w3359) -> (unsigned 8bit integer=w3358:u8[][])
            n2351 = call "IMAQ ArrayToImage"("Image Pixels (U8)"=w3358, "Image"=w3355) -> ("Image Out"=w3353:T2)  [unwired: 4 in, 5 out]
            n2352 = case shown="True" "Save Video" {
              tunnel: w3360 -> [_ w3418]
              tunnel: w3353 -> [_ w3417]
              frame False {
              }
              frame True {
                n2353 = call "IMAQ AVI Write Frame"("Image"=w3417, "Avi Refnum"=w3418) -> ()  [unwired: 2 in, 8 out]
              }
            }
            n2354 = case shown="True" "Save Image" {
              tunnel: w3358 -> [_ w3433]
              tunnel: w3357 -> [_ w3432]
              frame False {
              }
              frame True {
                n2355 = call <vilib>:"Flatten Pixmap.vi"("colors"=w3432, "8-bit pixmap"=w3433) -> ("image data"=w3439:T34)  [unwired: 4 in, 5 out]
                n2356 = call "Create new save file.vi"("Insert"="video_frame_" ("string"), "Ext"=".bmp" ("string"), "Index In"="Image Index") -> ("Path Out"=w3435:path, "Index Out"=w3440:dbl)
                n2357 = Increment(x=w3440) -> (x+1=w3434:dbl)
                n2358 = local write "Image Index"(w3434) -> ()
                n2359 = call <vilib>:"Write BMP File.vi"("image data"=w3439, "path to BMP file"=w3435) -> ()  [unwired: 1 in, 9 out]
              }
            }
            n2360 = case shown="True" "Target" {
              tunnel: w3353 -> [w3379 w3383]
              tunnel: [w3379 w3381] -> w3352
              frame False {
              }
              frame True {
                n2361 = local read "Target coordinates"() -> (w3380:cluster{"X1":dbl, "Y1":dbl, "X2":dbl, "Y2":dbl})
